vi "Teleop.vi"(10 "Match Info":T1={"Autonomous Elapsed Seconds"=0.0, "TeleOp Elapsed Seconds"=0.0, "Disabled Elapsed Seconds"=0.0, "Visited Autonomous"=FALSE, "Visited TeleOp"=FALSE, "Visited Disabled"=FALSE, "Autonomous Settings"={"Autonomous Style"=enum."Independent", "VI Refnum"=refnum}}, 11 "Call Context":T2) -> ()   [LabVIEW 2013]
doc: "This VI is called for each TeleOp packet received from the DS where the robot is not disabled. It is often used to read from the joysticks and update I/O or to update setpoints for timed control loops. It should complete and return within 20 milliseconds or it may miss DS packets."
uses:
  <vilib>/Rock Robotics/WPI/DriverStation/WPI_DriverStationDerivedRobotMode.ctl
  <vilib>/Rock Robotics/WPI/DriverStation/WPI_DriverStationMatch Info.ctl
  <vilib>/Rock Robotics/WPI/Solenoid/WPI_SolenoidValue.ctl
  Robot Global Data.vi
  <vilib>/Rock Robotics/WPI/Joystick/WPI_JoystickGetSetRefNum.vi
  <vilib>/Rock Robotics/WPI/RobotDrive/WPI_RobotDriveGetSetRefNum.vi
  <vilib>/Rock Robotics/WPI/Solenoid/WPI_SolenoidSetEnum.vi
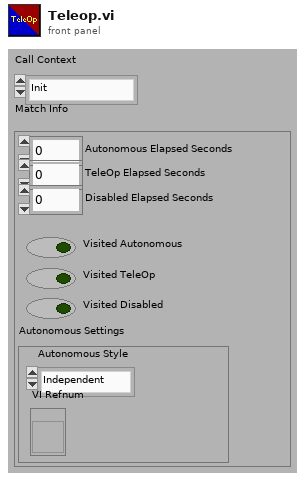
[diagram p1: front panel]
types:
  T1 = typedef "WPI_DriverStationMatch Info.ctl" = cluster{"Autonomous Elapsed Seconds":dbl, "TeleOp Elapsed Seconds":dbl, "Disabled Elapsed Seconds":dbl, "Visited Autonomous":bool, "Visited TeleOp":bool, "Visited Disabled":bool, "Autonomous Settings":cluster{"Autonomous Style":enum16{"Iterative", "Independent"}, "VI Refnum":refnum<vi>}}
  T2 = typedef "WPI_DriverStationDerivedRobotMode.ctl" = enum16{"Init", "Execute", "Stop"}
  T3 = typedef "WPI_JoystickDevRef.ctl" = cluster{"Device":T4}
  T4 = typedef "WPI_JoystickDeviceEnum.ctl" = enum16{"USB 1", "USB 2", "USB 3", "USB 4", "Kinect 1", "Kinect 2"}
  T5 = typedef "WPI_JoystickButtonState.ctl" = cluster{"Button 1":bool, "Button 2":bool, "Button 3":bool, "Button 4":bool, "Button 5":bool, "Button 6":bool, "Button 7":bool, "Button 8":bool, "Button 9":bool, "Button 10":bool, "Button 11":bool, "Button 12":bool}
  T6 = cluster{"axis 1 (x)":dbl, "axis 2 (y)":dbl, "axis 3 (throttle)":dbl, "axis 4":dbl, "axis 5":dbl, "axis 6":dbl}
  T7 = typedef "WPI_RobotDriveDevRef.ctl" = cluster{"DevStatus":errorcluster, "Motors[]":T8[], "Square Inputs":bool, "Max Output":dbl, "Isochronous":bool}
  T8 = typedef "WPI_MotorControlDeviceRef.ctl" = cluster{"DeviceStatus":errorcluster, "Type":enum16{"PWM", "CAN"}, "PWM":cluster{"Digital Module":T9, "PWM Channel":T10, "DeadBand":T11}, "CAN":cluster{"Device Number":u8, "Control Mode":T12, "Semaphore":T13, "Max Vout":dbl}, "Invert":bool, "TransformRef":T14, "InvTransformRef":T14}
  T9 = typedef "FPGA_TypedefDigitalModule.ctl" = enum16{"Digital Module 1", "Digital Module 2"}
  T10 = typedef "FPGA_DIOPWMChannel.ctl" = enum8{"PWM 1", "PWM 2", "PWM 3", "PWM 4", "PWM 5", "PWM 6", "PWM 7", "PWM 8", "PWM 9", "PWM 10", "Invalid"}
  T11 = typedef "WPI_PWMDeadband.ctl" = cluster{"Name":string, "maxPositivePwm":i32, "minPositivePwm":i32, "centerPwm":i32, "maxNegativePwm":i32, "minNegativePwm":i32, "angularRange":u16}
  T12 = typedef "WPI_CANJaguar_ControlMode.ctl" = enum8{"Percent VBus", "Current", "Speed", "Position", "Voltage"}
  T13 = typedef "Semaphore RefNum" = refnum<k1>
  T14 = typedef "WPI_PWMTransform_ConPane.ctl" = refnum<vi>
  T15 = typedef "WPI_SolenoidValue.ctl" = enum16{"Off", "On", "Forward", "Reverse"}
  T16 = typedef "WPI_SolenoidDevRef.ctl" = cluster{"DevStatus":errorcluster, "Solenoid Module":T17, "Forward Solenoid Channel":T18, "Reverse Solenoid Channel":T18}
  T17 = typedef "FPGA_TypedefSolenoidModule.ctl" = enum16{"Solenoid Module 1", "Solenoid Module 2"}
  T18 = typedef "WPI_SolenoidChannel.ctl" = enum8{"Solenoid 1", "Solenoid 2", "Solenoid 3", "Solenoid 4", "Solenoid 5", "Solenoid 6", "Solenoid 7", "Solenoid 8", "Invalid"}
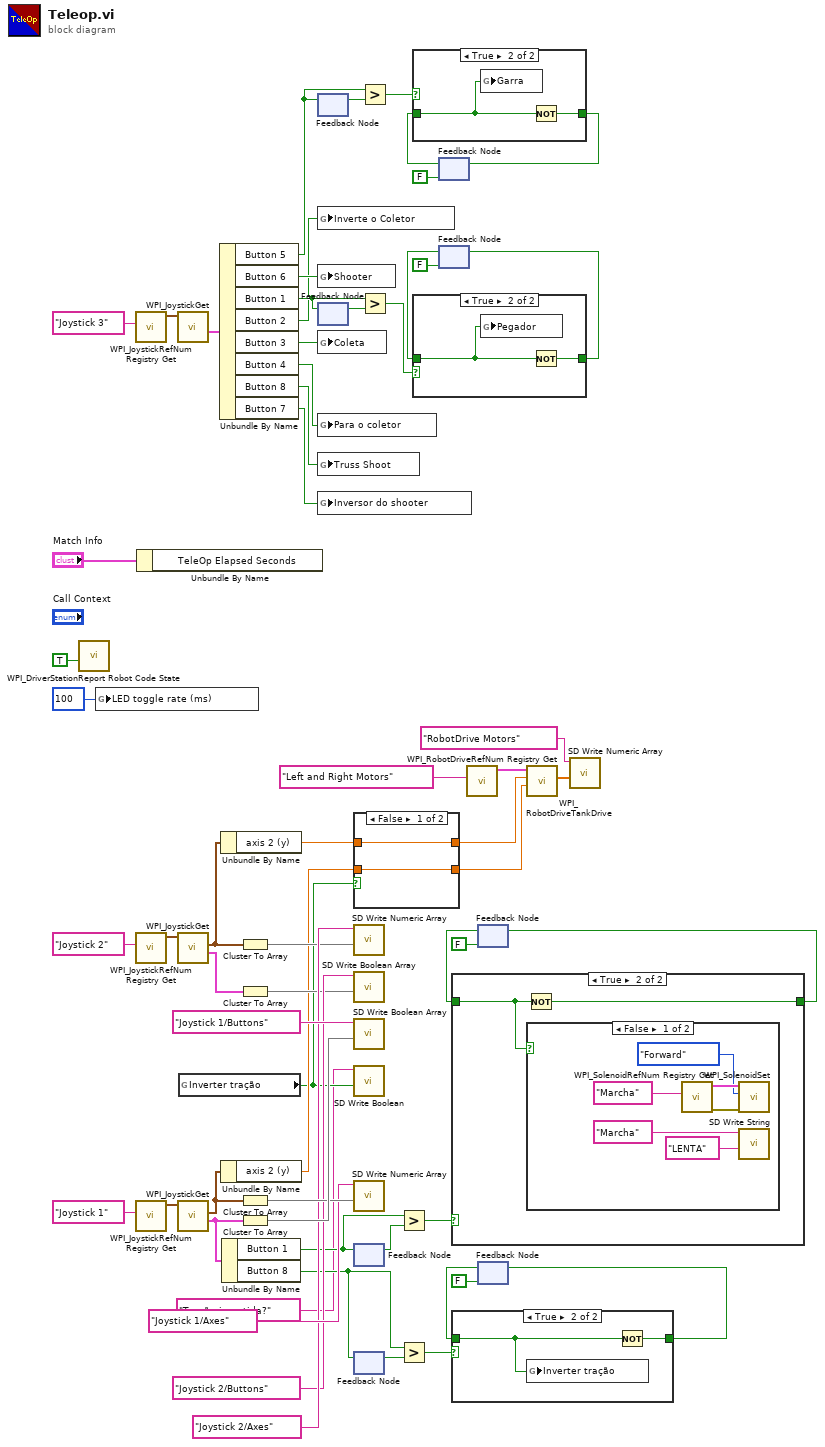
[diagram p0: block diagram]
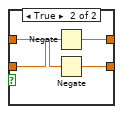
[diagram p3: hidden frame]
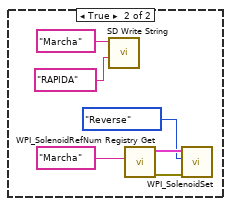
[diagram p7: hidden frame]
diagram:
  n1 = call <vilib>:"WPI_DriverStationReport Robot Code State.vi"("TeleOp"=TRUE ("Autonomous")) -> ()  [unwired: 10 in, 1 out]
  n2 = global write "Robot Global Data.vi" "LED toggle rate (ms)"(u32 100 ("LED ms toggle rate")) -> ()
  n3 = call <vilib>:"WPI_JoystickRefNum Registry Get.vi"("refnum name"="Joystick 3") -> ("JoystickDevRef"=w40:T3)  [unwired: 1 in, 9 out]
  n4 = call <vilib>:"WPI_JoystickRefNum Registry Get.vi"("refnum name"="Joystick 2") -> ("JoystickDevRef"=w45:T3)  [unwired: 1 in, 9 out]
  n5 = call <vilib>:"WPI_JoystickRefNum Registry Get.vi"("refnum name"="Joystick 1") -> ("JoystickDevRef"=w58:T3)  [unwired: 1 in, 9 out]
  n6 = Unbundle By Name("Match Info") -> ()  [unwired: 1 out]
  n7 = call <vilib>:"WPI_JoystickGet.vi"("JoystickDevRef"=w40) -> ("Buttons"=w38:T5)  [unwired: 1 in, 5 out]
  n8 = call <vilib>:"WPI_JoystickGet.vi"("JoystickDevRef"=w45) -> ("Buttons"=w41:T5, "Axes"=w46:T6)  [unwired: 1 in, 4 out]
  n9 = call <vilib>:"WPI_JoystickGet.vi"("JoystickDevRef"=w58) -> ("Buttons"=w26:T5, "Axes"=w53:T6)  [unwired: 1 in, 4 out]
  n10 = global read "Robot Global Data.vi" "Inverter tração"() -> (w7:bool)
  n11 = Unbundle By Name(w38) -> ("Button 5"=w23:bool, "Button 6"=w24:bool, "Button 1"=w27:bool, "Button 2"=w21:bool, "Button 3"=w20:bool, "Button 4"=w22:bool, "Button 8"=w19:bool, "Button 7"=w18:bool)
  n12 = Unbundle By Name(w46) -> ("axis 2 (y)"=w8:dbl)
  n13 = Unbundle By Name(w53) -> ("axis 2 (y)"=w9:dbl)
  n14 = Unbundle By Name(w26) -> ("Button 1"=w25:bool, "Button 8"=w12:bool)
  n15 = Cluster To Array(cluster=w46) -> (array=w47:dbl[])
  n16 = Cluster To Array(cluster=w41) -> (array=w42:bool[])
  n17 = Cluster To Array(cluster=w53) -> (array=w52:dbl[])
  n18 = Cluster To Array(cluster=w26) -> (array=w55:bool[])
  n19 = feedback #1() -> (w1:bool)  [unwired: 1 in]
  n20 = feedback-in #1(w23) -> ()
  n21 = global write "Robot Global Data.vi" "Inverte o Coletor"(w21) -> ()
  n22 = global write "Robot Global Data.vi" "Shooter"(w24) -> ()
  n23 = feedback #2() -> (w28:bool)  [unwired: 1 in]
  n24 = feedback-in #2(w27) -> ()
  n25 = global write "Robot Global Data.vi" "Coleta"(w20) -> ()
  n26 = global write "Robot Global Data.vi" "Para o coletor"(w22) -> ()
  n27 = global write "Robot Global Data.vi" "Truss Shoot"(w19) -> ()
  n28 = global write "Robot Global Data.vi" "Inversor do shooter"(w18) -> ()
  n29 = case shown="False" w7 {
    tunnel: w9 -> [w64 w67]
    tunnel: [w64 w66] -> w11
    tunnel: w8 -> [w63 w68]
    tunnel: [w63 w65] -> w10
    frame False {
    }
    frame True {
      n30 = Negate(x=w67) -> (-x=w65:dbl)
      n31 = Negate(x=w68) -> (-x=w66:dbl)
    }
  }
  n32 = call <vilib>:"SD Write Numeric Array.vi"("Numeric Array"=w47, "Name"="Joystick 2/Axes") -> ()  [unwired: 8 in, 2 out]
  n33 = call <vilib>:"SD Write Boolean Array.vi"("Boolean Array"=w42, "Name"="Joystick 2/Buttons") -> ()  [unwired: 8 in, 2 out]
  n34 = call <vilib>:"SD Write Boolean Array.vi"("Boolean Array"=w55, "Name"="Joystick 1/Buttons") -> ()  [unwired: 8 in, 2 out]
  n35 = call <vilib>:"SD Write Boolean.vi"("Boolean"=w7, "Name"="Tração invertida?") -> ()  [unwired: 8 in, 2 out]
  n36 = call <vilib>:"SD Write Numeric Array.vi"("Numeric Array"=w52, "Name"="Joystick 1/Axes") -> ()  [unwired: 8 in, 2 out]
  n37 = feedback-in #3(w25) -> ()
  n38 = feedback #3() -> (w37:bool)  [unwired: 1 in]
  n39 = feedback #4() -> (w15:bool)  [unwired: 1 in]
  n40 = feedback-in #4(w12) -> ()
  n41 = Greater?(x=w23, y=w1) -> (0:w5:bool)
  n42 = Greater?(x=w27, y=w28) -> (0:w29:bool)
  n43 = Greater?(x=w25, y=w37) -> (0:w36:bool)
  n44 = Greater?(x=w12, y=w15) -> (0:w17:bool)
  n45 = feedback #5(FALSE) -> (w4:bool)
  n46 = case shown="True" w5 {
    tunnel: w4 -> [w69 w70]
    tunnel: [w69 w71] -> w3
    frame False {
    }
    frame True {
      n47 = global write "Robot Global Data.vi" "Garra"(w70) -> ()
      n48 = Not(x=w70) -> (.not. x?=w71:bool)
    }
  }
  n49 = feedback-in #5(w3) -> ()
  n50 = feedback #6(FALSE) -> (w30:bool)
  n51 = case shown="True" w29 {
    tunnel: w30 -> [w72 w73]
    tunnel: [w72 w74] -> w31
    frame False {
    }
    frame True {
      n52 = global write "Robot Global Data.vi" "Pegador"(w73) -> ()
      n53 = Not(x=w73) -> (.not. x?=w74:bool)
    }
  }
  n54 = feedback-in #6(w31) -> ()
  n55 = call <vilib>:"WPI_RobotDriveRefNum Registry Get.vi"("refnum name"="Left and Right Motors") -> ("RobotDriveDevRef"=w60:T7)  [unwired: 1 in, 9 out]
  n56 = feedback #7(FALSE) -> (w34:bool)
  n57 = case shown="True" w36 {
    tunnel: w34 -> [w75 w76]
    tunnel: [w75 w77] -> w33
    frame False {
    }
    frame True {
      n58 = Not(x=w76) -> (.not. x?=w77:bool)
      n59 = case shown="False" w76 {
        frame False {
          n60 = call <vilib>:"WPI_SolenoidRefNum Registry Get.vi"("refnum name"="Marcha") -> ("error out"=w82:errorcluster, "SolenoidDevRef"=w83:T16)  [unwired: 9 in]
          n61 = call-poly <vilib>:"WPI_SolenoidSet.vi"("error in (no error)"=w82, "Value"=WPI_SolenoidValue."Forward", "SolenoidDevRef"=w83) -> ()  [unwired: 7 in, 2 out]
          n62 = call <vilib>:"SD Write String.vi"("String"="LENTA", "Name"="Marcha") -> ()  [unwired: 8 in, 2 out]
        }
        frame True {
          n63 = call <vilib>:"SD Write String.vi"("String"="RAPIDA", "Name"="Marcha") -> ()  [unwired: 8 in, 2 out]
          n64 = call <vilib>:"WPI_SolenoidRefNum Registry Get.vi"("refnum name"="Marcha") -> ("error out"=w87:errorcluster, "SolenoidDevRef"=w88:T16)  [unwired: 9 in]
          n65 = call-poly <vilib>:"WPI_SolenoidSet.vi"("error in (no error)"=w87, "Value"=WPI_SolenoidValue."Reverse", "SolenoidDevRef"=w88) -> ()  [unwired: 7 in, 2 out]
        }
      }
    }
  }
  n66 = feedback-in #7(w33) -> ()
  n67 = feedback #8(FALSE) -> (w13:bool)
  n68 = case shown="True" w17 {
    tunnel: w13 -> [w90 w91]
    tunnel: [w90 w92] -> w14
    frame False {
    }
    frame True {
      n69 = global write "Robot Global Data.vi" "Inverter tração"(w91) -> ()
      n70 = Not(x=w91) -> (.not. x?=w92:bool)
    }
  }
  n71 = feedback-in #8(w14) -> ()
  n72 = call <vilib>:"WPI_RobotDriveTankDrive.vi"("Right axis value"=w11, "Left axis value"=w10, "RobotDriveDevRef"=w60) -> ("Motor Values"=w49:dbl[])  [unwired: 6 in, 2 out]
  n73 = call <vilib>:"SD Write Numeric Array.vi"("Numeric Array"=w49, "Name"="RobotDrive Motors") -> ()  [unwired: 8 in, 2 out]
